vi "MoveToArena2.vi"   [LabVIEW 2016, in "Moving Motor.lvrbt"]
uses:
  Moving Motor.lvrbt
  <vilib>/NXT/Hardware/Plugins/Tetrix DC Motor/TetrixDCMotorAddress.ctl
  <vilib>/NXT/LegoClasses/BrickReference/BrickReference.lvclass
  <vilib>/NXT/Subs/LVHSConnector.ctl
  <vilib>/NXT/NXTIO Xnodes/NXTIONodeSubVIs/TETRIX IO Move DC Motors.vi
  <vilib>/NXT/NXTIO Xnodes/NXTIOXNode/NXTIO.xnode
  <vilib>/NXT/NXTIO Xnodes/AddressXNode/NXTIOAddress.xnode
  <vilib>/NXT/Block Support/NXT_InputPort.ctl
  <vilib>/NXT/Dual Mode Library/Sensors/EV3_Color_Color.vi
  <vilib>/NXT/NXTIO Xnodes/NXTIONodeSubVIs/TETRIX IO Stop DC Motors.vi
types:
  T1 = typedef "NXT_InputPort.ctl" = u32
  T2 = typedef "TetrixDCMotorAddress.ctl" = i32
  T3 = typedef "LVHSConnector.ctl" = refnum<class "BrickReference.lvclass">
  T4 = cluster{"TetrixDCMotor":T2, "TetrixDCMotor 2":T2}
  T5 = typedef "ColorSensorColors.ctl" = enum16{"No Color", "Black", "Blue", "Green", "Yellow", "Red", "White", "Brown"}
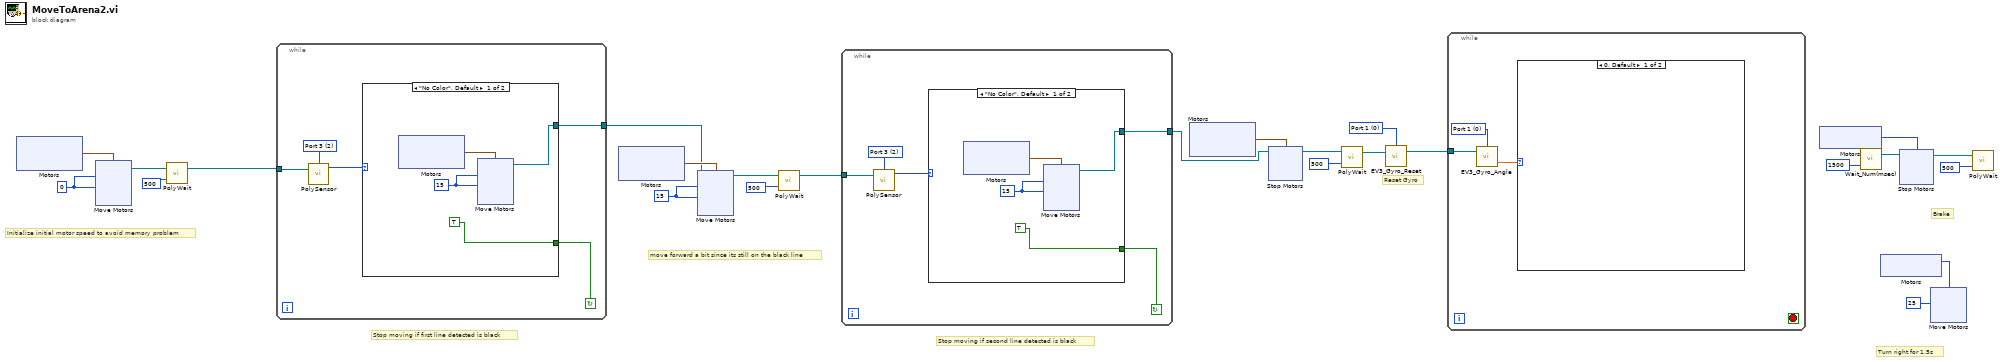
[diagram p0: block diagram]
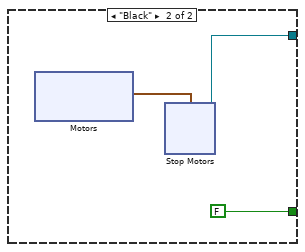
[diagram p3: hidden frame]
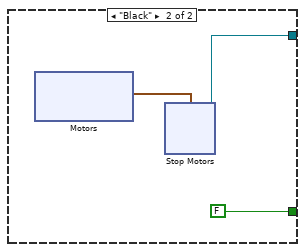
[diagram p4: hidden frame]
diagram:
  w2 = T1 0 items=["Port 1", "Port 2", "Port 3", "Port 4"] ("Port (Port 1)")
  w21 = 15
  w24 = 0
  # "Reset Gyro"
  # "Turn right for 1.5s"
  # "Brake"
  # "move forward a bit since its still on the black line"
  # "Stop moving if second line detected is black"
  # "Stop moving if first line detected is black"
  # "Initialize initial motor speed to avoid memory problem"
  n1 = xnode "Motors"() -> ("Motor"=w25:cluster{"TetrixDCMotor":T2, "TetrixDCMotor":T2})
  n2 = xnode "Move Motors"("Power/Speed 2"=w24, "Power/Speed 1"=w24, "Motors"=w25) -> ("NXT/EV3"=w22:T3)  [unwired: 1 in]
  n3 = call-poly <vilib>:"PolyWait.vi"("Time (100 msec)"=500, "NXT/EV3"=w22) -> ("NXT/EV3"=w11:T3)  [unwired: 2 in]
  n4 = while {
    tunnel: w11 -> [w29]
    tunnel: [w26] -> w19
    stop <- w27 continue-if-true
    w30 = T1 2 items=["Port 1", "Port 2", "Port 3", "Port 4"] ("Port (Port 1)")
    n5 = call-poly <vilib>:"PolySensor.vi"("NXT/EV3"=w29, "Port (Port 1)"=w30) -> ("Detected Color"=w28:T5)  [unwired: 1 in, 1 out]
    n6 = case shown="\"No Color\", Default" w28 {
      tunnel: [TRUE FALSE] -> w27
      tunnel: [w31 w44] -> w26
      frame "No Color", Default {
        w34 = 15
        n7 = xnode "Motors"() -> ("Motor"=w33:cluster{"TetrixDCMotor":T2, "TetrixDCMotor":T2})
        n8 = xnode "Move Motors"("Power/Speed 2"=w34, "Power/Speed 1"=w34, "Motors"=w33) -> ("NXT/EV3"=w31:T3)  [unwired: 1 in]
      }
      frame "Black" {
        n9 = xnode "Motors"() -> ("Motor"=w46:cluster{"TetrixDCMotor":T2, "TetrixDCMotor":T2})
        n10 = xnode "Stop Motors"("Motors"=w46) -> ("NXT/EV3"=w44:T3)  [unwired: 1 in]
      }
    }
  }
  n11 = xnode "Motors"() -> ("Motor"=w20:cluster{"TetrixDCMotor":T2, "TetrixDCMotor":T2})
  n12 = xnode "Move Motors"("Power/Speed 2"=w21, "Power/Speed 1"=w21, "Motors"=w20, "NXT/EV3"=w19) -> ("NXT/EV3"=w17:T3)
  n13 = call-poly <vilib>:"PolyWait.vi"("Time (100 msec)"=500, "NXT/EV3"=w17) -> ("NXT/EV3"=w16:T3)  [unwired: 2 in]
  n14 = while {
    tunnel: w16 -> [w56]
    tunnel: [w53] -> w12
    stop <- w54 continue-if-true
    w57 = T1 2 items=["Port 1", "Port 2", "Port 3", "Port 4"] ("Port (Port 1)")
    n15 = call-poly <vilib>:"PolySensor.vi"("NXT/EV3"=w56, "Port (Port 1)"=w57) -> ("Detected Color"=w55:T5)  [unwired: 1 in, 1 out]
    n16 = case shown="\"No Color\", Default" w55 {
      tunnel: [TRUE FALSE] -> w54
      tunnel: [w58 w71] -> w53
      frame "No Color", Default {
        w61 = 15
        n17 = xnode "Motors"() -> ("Motor"=w60:cluster{"TetrixDCMotor":T2, "TetrixDCMotor":T2})
        n18 = xnode "Move Motors"("Power/Speed 2"=w61, "Power/Speed 1"=w61, "Motors"=w60) -> ("NXT/EV3"=w58:T3)  [unwired: 1 in]
      }
      frame "Black" {
        n19 = xnode "Motors"() -> ("Motor"=w73:cluster{"TetrixDCMotor":T2, "TetrixDCMotor":T2})
        n20 = xnode "Stop Motors"("Motors"=w73) -> ("NXT/EV3"=w71:T3)  [unwired: 1 in]
      }
    }
  }
  n21 = xnode "Motors"() -> ("Motor"=w15:cluster{"TetrixDCMotor":T2, "TetrixDCMotor":T2})
  n22 = xnode "Stop Motors"("Motors"=w15, "NXT/EV3"=w12) -> ("NXT/EV3"=w14:T3)
  n23 = call-poly <vilib>:"PolyWait.vi"("Time (100 msec)"=500, "NXT/EV3"=w14) -> ("NXT/EV3"=w3:T3)  [unwired: 2 in]
  n24 = call <vilib>:"EV3_Gyro_Reset.vi"("NXT/EV3"=w3, "Port (Port 1)"=w2) -> ("NXT/EV3"=w1:T3)  [unwired: 2 in]
  n25 = while {
    tunnel: w1 -> [w82]
    stop <- _ stop-if-true
    w80 = T1 0 items=["Port 1", "Port 2", "Port 3", "Port 4"] ("Port (Port 1)")
    n26 = call <vilib>:"EV3_Gyro_Angle.vi"("NXT/EV3"=w82, "Port (Port 1)"=w80) -> ("Degrees"=w81:sgl)  [unwired: 1 in, 1 out]
    n27 = case shown="0, Default" w81 {
      frame 0, Default {
      }
      frame 1 {
      }
    }
  }
  n28 = xnode "Motors"() -> ("Motor"=w6:T2)
  n29 = call <vilib>:"Wait_Num(msec).vi"("Time (100 msec)"=1500) -> ("NXT/EV3"=w7:T3)  [unwired: 3 in]
  n30 = xnode "Motors"() -> ("Motor"=w4:T2)
  n31 = xnode "Stop Motors"("Motors"=w6, "NXT/EV3"=w7) -> ("NXT/EV3"=w9:T3)
  n32 = xnode "Move Motors"("Power/Speed 1"=25, "Motors"=w4) -> ()  [unwired: 1 in, 1 out]
  n33 = call-poly <vilib>:"PolyWait.vi"("Time (100 msec)"=500, "NXT/EV3"=w9) -> ()  [unwired: 2 in, 1 out]
